vi "FTW-Listener-Wait On Connection.vi"(0 "FTW-Listener-TCP In":refnum<class "FTW-Listener-TCP.lvclass">, 11 "error in":errorcluster) -> (4 "FTW-Listener-TCP Out":refnum<class "FTW-Listener-TCP.lvclass">, 6 "Endpoint":refnum<class "FTW-Endpoint.lvclass">, 15 "error out":errorcluster)   [LabVIEW 2013, in "FTW-Listener-TCP.lvclass"]
uses:
  FTW-Listener-TCP.lvclass
  Endpoint/FTW-Endpoint.lvclass
  TCP/FTW-Endpoint-TCP.lvclass
  FTW-Listener-TCP.lvclass/FTW-Listener-TCP.ctl
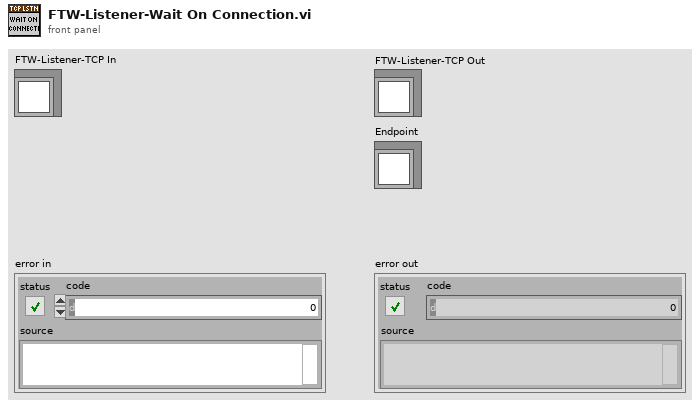
[diagram p1: front panel]
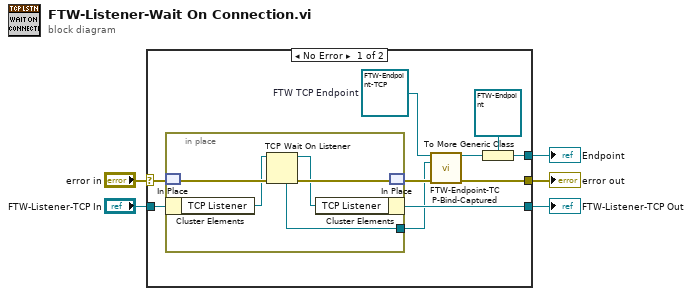
[diagram p0: block diagram]
diagram:
  n1 = case shown="No Error" "error in" {
    selector: "error in" -> [w14 w22]
    tunnel: [w11 w22] -> w4
    tunnel: [w15 w21] -> w3
    tunnel: "FTW-Listener-TCP In" -> [w13 w21]
    tunnel: [w9 _] -> w1
    frame No Error {
      w7 = refnum<class "FTW-Endpoint-TCP.lvclass"> refnum  # FTW TCP Endpoint
      n2 = in-place {
        in-place-border: [w16] -> w6
        n3 = in-place-match #1(w14) -> (w20:errorcluster)
        n4 = in-place-cluster #2(w13) -> ("TCP Listener"=w17:refnum<k5>)
        n5 = TCP Wait On Listener(8:w20, 11:w17) -> (0:w19:errorcluster, 3:w18:refnum<k5>, 4:w16:refnum<k5>)  [unwired: 2 in, 2 out]
        n6 = in-place-cluster #2("TCP Listener"=w18) -> (w15:refnum<class "FTW-Listener-TCP.lvclass">)
        n7 = in-place-match #1(w19) -> (w12:errorcluster)
      }
      n8 = call-dynamic "FTW-Endpoint-TCP-Bind-Captured.vi"("FTW Endpoint"=w7, "Connection"=w6, "error in"=w12) -> ("FTW Endpoint out"=w10:refnum<class "FTW-Endpoint-TCP.lvclass">, "error out"=w11:errorcluster)  [unwired: 9 in, 2 out]
      n9 = To More Generic Class(target class=refnum<class "FTW-Endpoint.lvclass"> refnum ("FTW Endpoint"), reference=w10) -> (generic class reference=w9:refnum<class "FTW-Endpoint.lvclass">)
    }
    frame Error {
    }
  }
  "FTW-Listener-TCP Out" <- w3
  "error out" <- w4
  "Endpoint" <- w1
